vi "keyscale.vi"(10 "project-param in":T2, 11 "Scales":T1) -> (1 "project-param out 2":T2, 2 "Array":string[](array[string]), 3 "Scale Notes":bool[](array[boolean]))   [LabVIEW 2019]
uses:
  Project Parameters.ctl
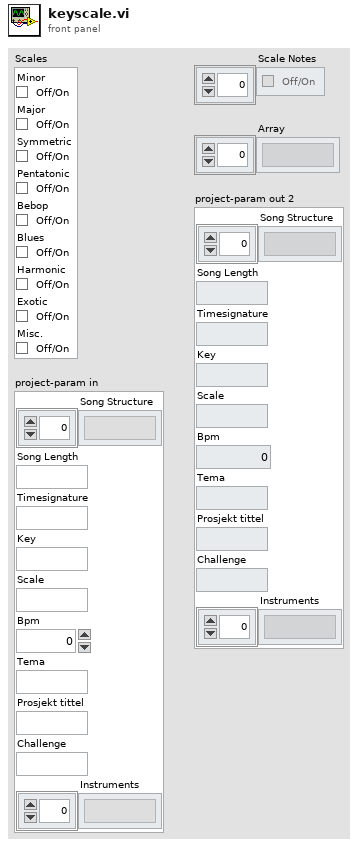
[diagram p1: front panel]
types:
  T1 = cluster{"Minor":bool, "Major":bool, "Symmetric":bool, "Pentatonic":bool, "Bebop":bool, "Blues":bool, "Harmonic":bool, "Exotic":bool, "Misc.":bool}
  T2 = typedef "Project Parameters.ctl" = cluster{"Song Structure":string[], "Song Length":string, "Timesignature":string, "Key":string, "Scale":string, "Bpm":i32, "Tema":string, "Prosjekt tittel":string, "Challenge":string, "Instruments":string[]}
  T3 = cluster{"Keys":string[], "Melodic Minor Scales":string[], "Minor Tones":bool[][], "Major Scales":string[], "Major Tones":bool[][], "Symmetric Scales":string[], "Symmetric Tones":bool[][], "Pentatonic Scales":string[], "Pentatonic Tones":bool[][], "Blues Scale":string[], "Blues Tones":bool[][], "Bebop Scale":string[], "Bebop Tones":bool[][], "Harmonic Scales":string[], "Harmonic Tones":bool[][], "Exotic Scales":string[], "Exotic Tones":bool[][], "Miscellaneous Scales":string[], "Miscellaneous Tones":bool[][]}
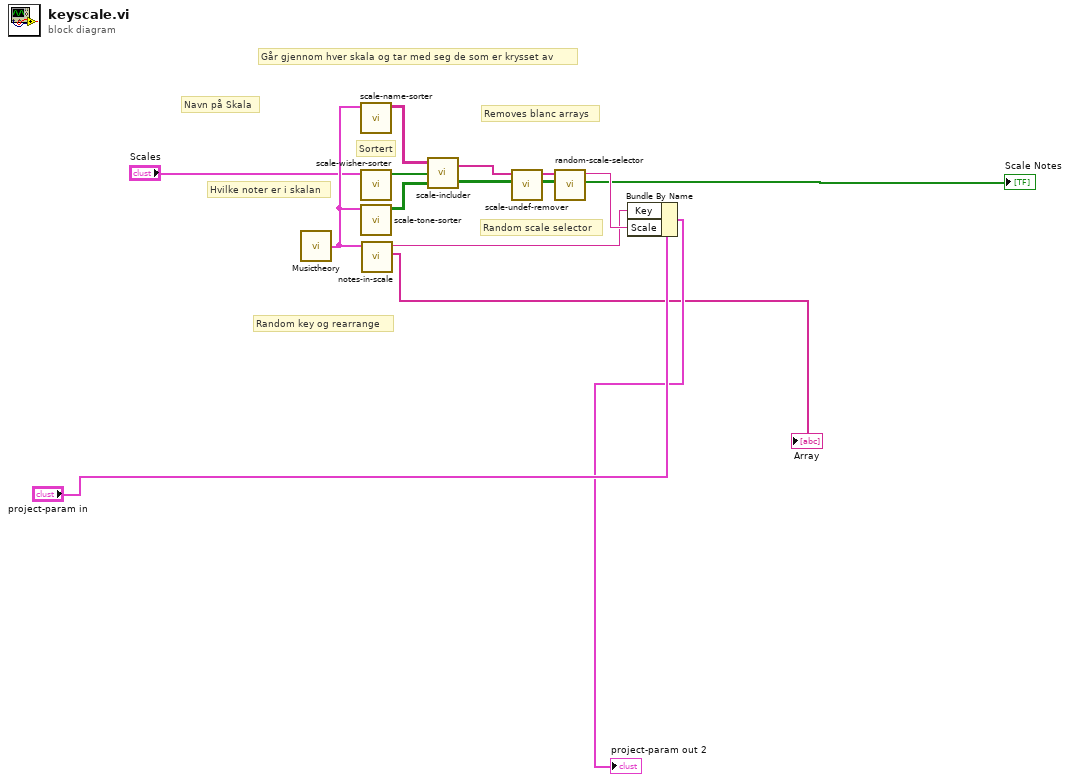
[diagram p0: block diagram]
diagram:
  # "Random scale selector"
  # "Random key og rearrange"
  # "Removes blanc arrays"
  # "Sortert"
  # "Navn på Skala"
  # "Hvilke noter er i skalan"
  # "Går gjennom hver skala og tar med seg de som er krysset av"
  n1 = call "Musictheory.vi"() -> ("Cluster"=w5:T3)  [unwired: 2 in]
  n2 = call "scale-name-sorter.vi"("Cluster"=w5) -> ("Array"=w9:string[][])  [unwired: 10 in]
  n3 = call "scale-wisher-sorter.vi"("Scales"="Scales") -> ("Scale notes"=w11:bool[])  [unwired: 10 in]
  n4 = call "scale-tone-sorter.vi"("Cluster"=w5) -> ("Array"=w10:bool[][][])  [unwired: 10 in]
  n5 = call "notes-in-scale.vi"("Cluster"=w5) -> ("Array"=→"Array":string[], "String"=w12:string)  [unwired: 9 in]
  n6 = call "scale-includer.vi"("All Scale Notes"=w10, "Selected scales"=w11, "All Scale Names"=w9) -> ("Selected Scale Notes"=w8:bool[][], "Selected Scale Names"=w1:string[])
  n7 = call "scale-undef-remover.vi"("Scalenotes Undef"=w8, "Scalename undef"=w1) -> ("Scale Notes"=w3:bool[][], "Scale Names"=w2:string[])  [unwired: 8 in]
  n8 = call "random-scale-selector.vi"("Scale Notes"=w3, "Scale Names"=w2) -> ("Scale Notes"=→"Scale Notes":bool[], "Scale Name"=w13:string)  [unwired: 8 in]
  n9 = Bundle By Name(cluster="project-param in", "Key"=w12, "Scale"=w13) -> (→"project-param out 2":T2)
